vi "SelectPressureUnit Example.vi"() -> ()   [LabVIEW 2019]
uses:
  BrooksDLL.dll
panel:
  in  "Pressure Unit Code":u8(ring) items=["In of H2O", "In of Hg", "Ft of H2O", "PSI", "Bar", "mBar", "Pascals", "kiloPascals", "Torr", "Std Atmosphere", "kg/cm2", "mTorr", "mm Hg", "gr/cm2", "cm of H2O"]
  out "S2 String":string
  out "S1 String":string
  out "S2":u8 format="%.0x"
  out "S1":u8 format="%.0x"
  out "Function Output Comment":string
  out "output param":i32
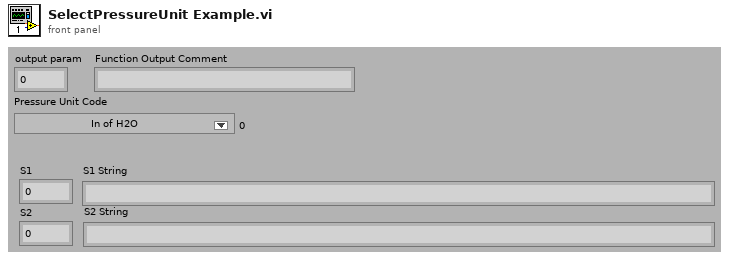
[diagram p1: front panel]
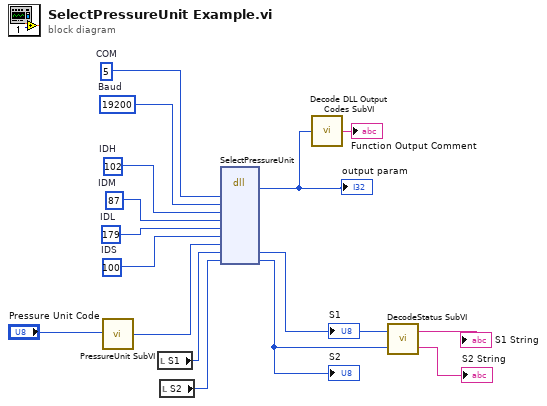
[diagram p0: block diagram]
diagram:
  w11 = u8 100  # IDS
  w12 = u8 179  # IDL
  w13 = u8 87  # IDM
  w14 = u8 102  # IDH
  w15 = 19200  # Baud
  w16 = 5  # COM
  n1 = call "PressureUnit SubVI.vi"("Flow Unit"="Pressure Unit Code") -> ("FlowUnit"=w5:u8)
  n2 = local read "S1"() -> (w4:u8)
  n3 = local read "S2"() -> (w3:u8)
  n4 = dll-call lib="G:/Developpement_de_Programmes/Programmes/Controle de pression/164J027_AD/Brooks DLL 1.0.1.0 32bit/Brooks DLL 1.0.1.0 Release 10032016/S Protocol/BrooksDLL.dll" fn="SelectPressureUnit"("COM"=w16, "Baud"=w15, "IDH"=w14, "IDM"=w13, "IDL"=w12, "IDS"=w11, "PressureUnitCode"=w5, "S1"=w4, "S2"=w3) -> (w10:i32, "S1"=w2:u8, "S2"=w1:u8)  [unwired: 10 in, 2 out]
  "output param" <- w10
  "S1" <- w2
  "S2" <- w1
  n5 = call "Decode DLL Output Codes SubVI.vi"("Numeric"=w10) -> ("Function Output Comment"=→"Function Output Comment":string)
  n6 = call "DecodeStatus SubVI.vi"("S2"=w1, "S1"=w2) -> ("S2 String"=→"S2 String":string, "S1 String"=→"S1 String":string)
